vi "Setup SSR.vi"(0 "reference in":refnum<class "SSR.lvclass">, 3 "Module Names (NI-MAX Alias)":string[](array[string])=["SSR-8CH"], 4 "Number of Channels Per Module":u32[](array[numeric])=[8], 5 "error in (no error)":errorcluster) -> (14 "reference out":refnum<class "SSR.lvclass">, 19 "error out":errorcluster)   [LabVIEW 2017, in "SSR.lvclass"]
uses:
  SSR.lvclass
  <vilib>/DAQmx/create/channels.llb/DAQmx Create Channel (DO-Digital Output).vi
  <resource>/objmgr/daqmx.rc
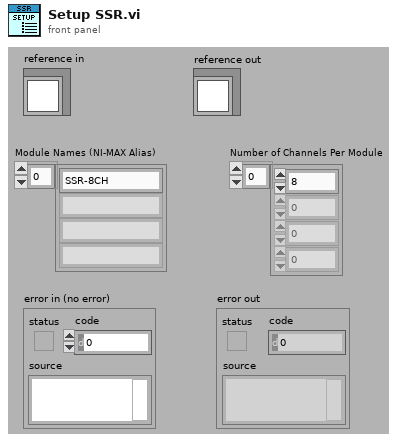
[diagram p1: front panel]
types:
  T1 = typedef "SSR.lvclass/ObjectAttributes.ctl" = cluster{"SSR Task":refnum<k21>, "SSR On/Off Status":bool, "Number of SSR Modules":u32, "Number of Total SSR Channels":u32, "SSR Module Names (NI-Max Name)":string[], "Number of Channels Per SSR Module":i32[], "SSR Status":bool[], "SSR Status to Set":bool[], "SSR VI Reference":refnum<vi>}
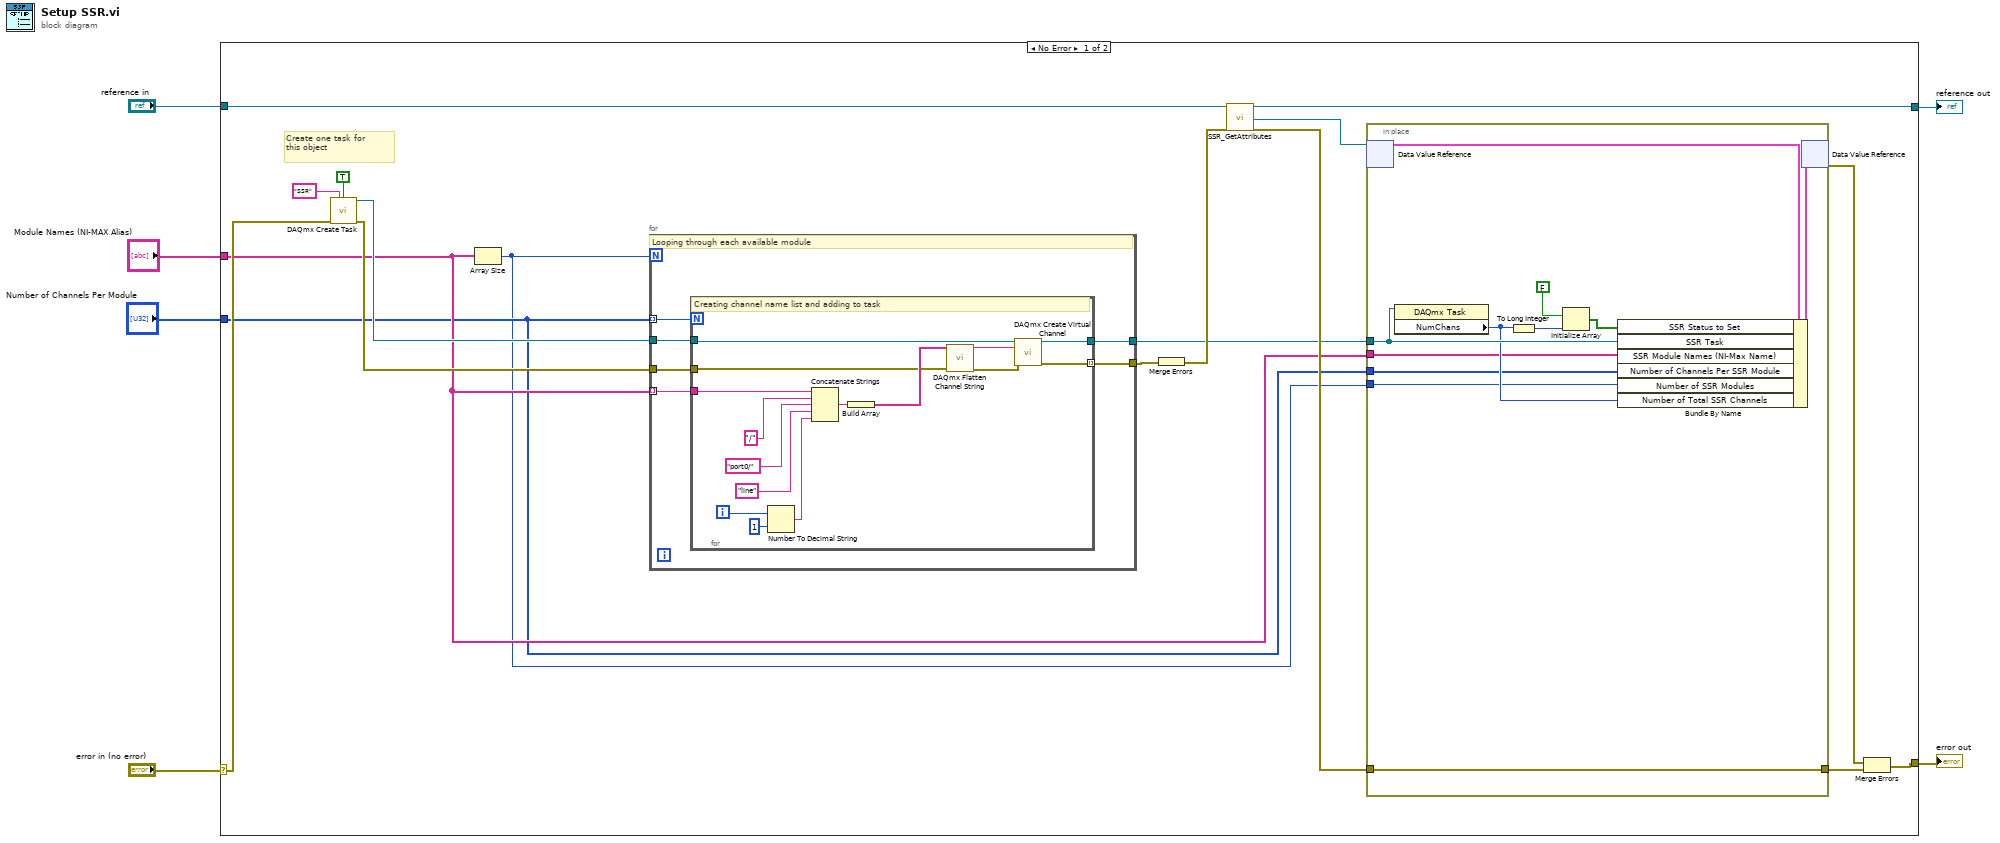
[diagram p0: block diagram]
diagram:
  n1 = case shown="No Error" "error in (no error)" {
    selector: "error in (no error)" -> [w11 w58]
    tunnel: [w21 w58] -> w5
    tunnel: [w22 w57] -> w3
    tunnel: "reference in" -> [w24 w57]
    tunnel: "Module Names (NI-MAX Alias)" -> [w9 _]
    tunnel: "Number of Channels Per Module" -> [w8 _]
    frame No Error {
      # "Create one task for \nthis object"
      n2 = call <vilib>:"DAQmx Create Task.vi"("new task name"="SSR", "auto cleanup"=TRUE, "error in"=w11) -> ("task out"=w13:refnum<k21>, "error out"=w17:errorcluster)  [unwired: 11 in]
      n3 = Array Size(array=w9) -> (size(s)=w7:i32)
      n4 = for {
        N: w7 -> [_]
        tunnel: w17 -> [w30]
        tunnel: [w29] -> w14
        tunnel: [w28] -> w10
        tunnel: w13 -> [w27]
        tunnel: w8 -> [w26] mode=indexing
        tunnel: w9 -> [w25] mode=indexing
        # "Looping through each available module"
        n5 = for {
          N: w26 -> [_]
          tunnel: w27 -> [w39]
          tunnel: [w38] -> w28
          tunnel: w30 -> [w34]
          tunnel: [w33] -> w29 mode=indexing
          tunnel: w25 -> [w32]
          i -> [w31]
          # "Creating channel name list and adding to task"
          n6 = Number To Decimal String(number=w31, width (-)=i16 1) -> (decimal integer string=w42:string)
          n7 = Concatenate Strings(w32, "/", "port0/", "line", w42) -> (w37:string)
          n8 = Build Array(w37) -> (w36:string[])
          n9 = call <vilib>:"DAQmx Flatten Channel String.vi"("names in"=w36, "error in"=w34) -> ("names out"=w40:string, "error out"=w41:errorcluster)  [unwired: 12 in]
          n10 = call-poly <vilib>:"DAQmx Create Virtual Channel.vi"("task in"=w39, "lines"=w40, "error in"=w41) -> ("task out"=w38:refnum<k21>, "error out"=w33:errorcluster)  [unwired: 11 in]
        }
      }
      n11 = Merge Errors(w14) -> (w12:errorcluster)
      n12 = call "SSR_GetAttributes.vi"("reference in"=w24, "error in (no error)"=w12) -> ("reference out"=w22:refnum<class "SSR.lvclass">, "DataRef"=w20:refnum<data-value>, "error out"=w19:errorcluster)  [unwired: 14 in, 1 out]
      n13 = in-place {
        in-place-border: w19 -> [w54]
        in-place-border: [w54] -> w18
        in-place-border: w10 -> [w51]
        in-place-border: w9 -> [w48]
        in-place-border: w8 -> [w47]
        in-place-border: w7 -> [w46]
        n14 = in-place-dvr #1(w20) -> (w55:T1)  [unwired: 1 out]
        n15 = property class="DAQmx Task"(reference=w51) -> ("NumChans"=w49:u32)  [unwired: 1 in, 2 out]
        n16 = To Long Integer(number=w49) -> (32bit integer=w52:i32)
        n17 = Initialize Array(FALSE, w52) -> (w50:bool[])
        n18 = Bundle By Name(cluster=w55, "SSR Status to Set"=w50, "SSR Task"=w51, "SSR Module Names (NI-Max Name)"=w48, "Number of Channels Per SSR Module"=w47, "Number of SSR Modules"=w46, "Number of Total SSR Channels"=w49) -> (w56:T1)
        n19 = in-place-dvr #1(w56) -> (w23:errorcluster)  [unwired: 1 out]
      }
      n20 = Merge Errors(w23, w18) -> (w21:errorcluster)
    }
    frame Error {
    }
  }
  "error out" <- w5
  "reference out" <- w3
